vi "Read Description.vi"(11 "Soy in":refnum<class "Soy.lvclass">) -> (2 "Description":string, 3 "Soy out":refnum<class "Soy.lvclass">)   [LabVIEW 2020, in "Soy.lvclass"]
uses:
  Soy.lvclass
  Soy.lvclass/Soy.ctl
  Beverage.lvclass
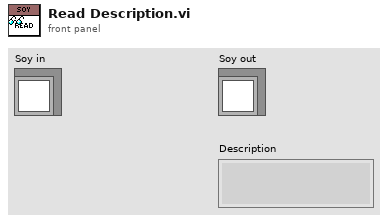
[diagram p1: front panel]
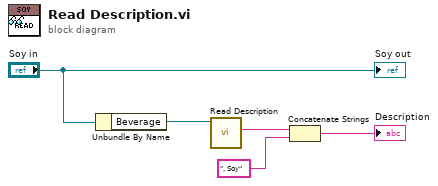
[diagram p0: block diagram]
diagram:
  n1 = Unbundle By Name("Soy in") -> ("Beverage"=w4:refnum<class "Beverage.lvclass">)
  n2 = call-dynamic "Read Description.vi"("Beverage in"=w4) -> ("Description"=w3:string)  [unwired: 9 in, 1 out]
  n3 = Concatenate Strings(w3, ", Soy" ("string")) -> (→"Description":string)
  "Soy out" <- "Soy in"
